vi "PH_Sound.Play Song.vi"(0 "i ref in":refnum<vi>, 2 "Song":cluster{"Tone":dbl, "Beats":i32}[](array[cluster]), 5 "error in (no error)":errorcluster) -> (14 "i ref out":refnum<vi>, 19 "error out":errorcluster)   [LabVIEW 2014, in "PH_Sound.lvlib"]
doc: "This VI play the connected Song"
uses:
  PH_Sound.lvlib
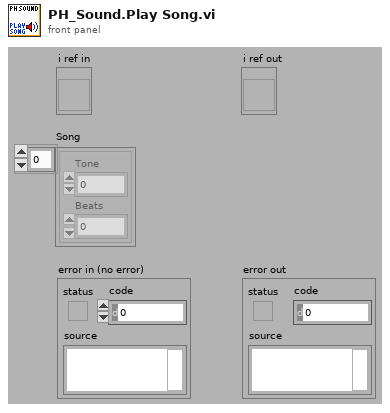
[diagram p1: front panel]
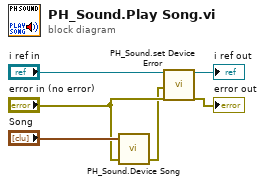
[diagram p0: block diagram]
diagram:
  n1 = call "PH_Sound.Device Song.vi"("error in (no error)"="error in (no error)", "Song"="Song") -> ("error out"=w1:errorcluster)  [unwired: 3 in]
  n2 = call "PH_Sound.set Device Error.vi"("VI in"="i ref in", "Device error"=w1, "error in"="error in (no error)") -> ("VI out"=→"i ref out":refnum<vi>, "error out"=→"error out":errorcluster)  [unwired: 15 in]
